vi "Process Data and Plot.vi"(8 "error in (no error)":errorcluster, 9 "Pressure":dbl[](array[numeric]), 10 "Graph":dbl[](array[numeric]), 11 "WaveformGraph in":refnum<vi>) -> (0 "error out":errorcluster)   [LabVIEW 2013, in "main.lvlib"]
uses:
  main.lvlib
  Controls/Enum Variables.ctl
  <vilib>/Analysis/baseanly.llb/Mean (DBL).vi
  <vilib>/Analysis/NI_AALBase.lvlib
panel:
  out "Waveform Graph":dbl[](graph)
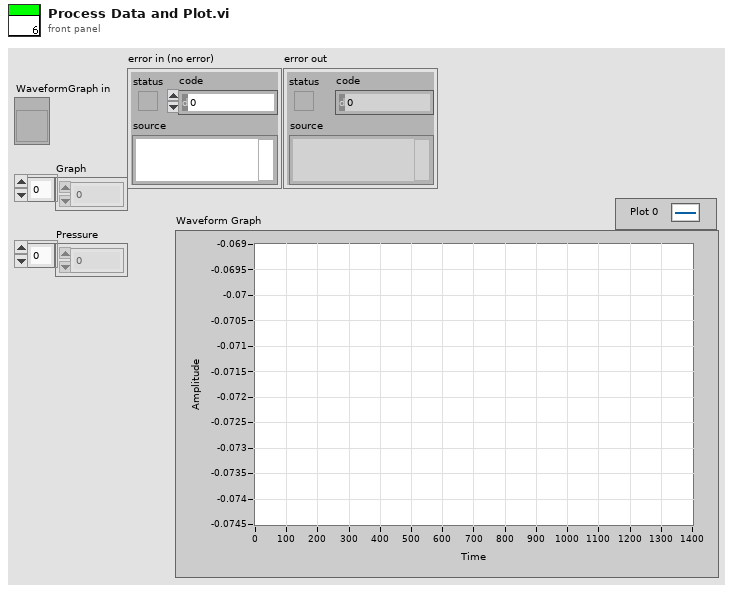
[diagram p1: front panel]
types:
  T1 = typedef "main.lvlib/Enum Variables.ctl" = enum16{"SetAcqFilter", "GetAcqFilter", "Set Filter", "Get Filter", "Set Height", "Get Height", "Set Recorded Height", "Get Recorded Height", "Set Blue Pressure", "Get Blue Pressure", "Set Red Pressure", "Get Red Pressure", "Init", "Reset Pressure", "Set Red Cursors", "Get Red Cursors", "Set Blue Cursors", "Get Blue Cursors", "Set Language", "Get Language", "Set Active Graphs", "Get ActiveGraphs", "Set Method", "Get Method", "Set Encryption", "Get Encryption", "Set ExcelVersion", "Get ExcelVersion", "Set DICOM Avail", "Get DICOM Avail", "Set DICOM Encode", "Get DICOM Encode", "Set JournalExport", "Get JournalExport", "Set Sequence", "Get Sequence", "Set DAQ Connected", "Get DAQ Connected", "Set Current Graph", "Get Current Graph", "Set General Settings", "Get Hyphenation", "Set Arm Calc Method", "Get Arm Calc Method", "Set Dicom Tags", "Get Dicom Tags", "Set BT Serial", "Get BT Serial", "Set BT Accepted Serials", "Get BT Accepted Serials", "Get BT License", "Set BT License"}
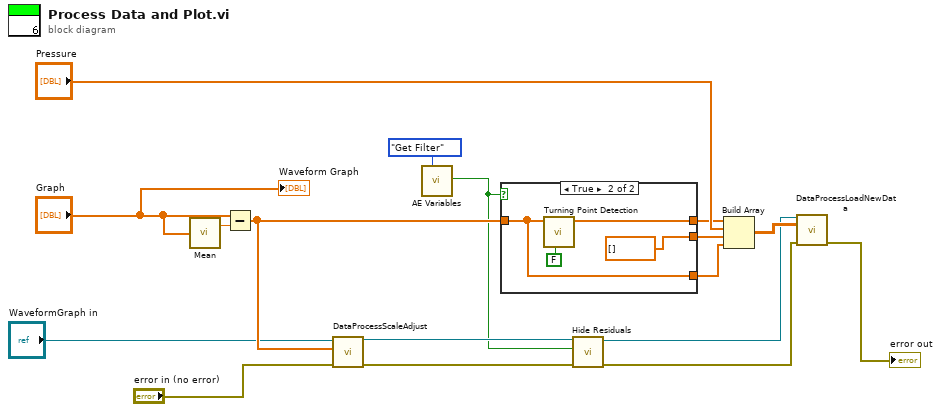
[diagram p0: block diagram]
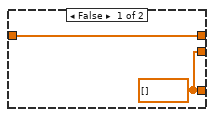
[diagram p2: hidden frame]
diagram:
  n1 = call-poly <vilib>:"Mean.vi"("X"="Graph") -> ("mean"=w12:dbl)  [unwired: 1 out]
  n2 = Subtract(x="Graph", y=w12) -> (x-y=w15:dbl[])
  n3 = call "DataProcessScaleAdjust.vi"("error in (no error)"="error in (no error)", 10:"Graph"=w15, 11:"Graph"="WaveformGraph in") -> ("error out"=w5:errorcluster, "reference out"=w6:refnum<vi>)  [unwired: 7 in]
  n4 = call "AE Variables.vi"("Action"=Enum_Variables."Get Filter") -> ("BooleanOut"=w2:bool)  [unwired: 11 in, 7 out]
  n5 = case shown="True" w2 {
    tunnel: w15 -> [w19 w21]
    tunnel: [w19 w22] -> w9
    tunnel: [w18 w21] -> w8
    tunnel: [w18 dbl[] []] -> w7
    frame False {
      w18 = dbl[] []
    }
    frame True {
      n6 = call "Turning Point Detection.vi"("Detect Points?"=FALSE, "Input"=w21) -> ("Best BSpline Fit"=w22:dbl[])  [unwired: 8 in, 1 out]
    }
  }
  n7 = call "Hide Residuals.vi"("error in (no error)"=w5, "Residuals"=w2, "WaveformGraph in"=w6) -> ("error out"=w4:errorcluster, "WaveformGraph out"=w3:refnum<vi>)  [unwired: 7 in]
  n8 = Build Array(w9, "Pressure", w7, w8) -> (w17:dbl[][])
  n9 = call "DataProcessLoadNewData.vi"("Graph"=w3, "Data"=w17, "error in (no error)"=w4) -> ("error out"=→"error out":errorcluster)  [unwired: 11 in, 1 out]
  "Waveform Graph" <- "Graph"
